vi "Main FPGA 8-axis for WPC.vi"() -> ()   [LabVIEW 2015]
uses:
  <vilib>/Motion/MotorControl/_s/nism.interpretControlRegister.stateTransition.ctl
  <vilib>/Platform/TimedLoop/XDataNode/timing_clust.ctl
  <vilib>/Platform/TimedLoop/XDataNode/nitl_modes.ctl
  <vilib>/Platform/TimedLoop/XDataNode/wakeup.ctl
  <vilib>/rvi/Emulation/niFpgaGetClockAttributes.vi
  <vilib>/rvi/Emulation/niFpgaSctlEmulationGetInTimedLoop.vi
  <vilib>/rvi/Emulation/niFpgaEmulationReportErrorSimple.vi
  Global FPGA 8-axis.vi
  <vilib>/Motion/MotorControl/_s/nism.interpretControlRegister.indexed.vi
  <vilib>/rvi/Emulation/niFpgaProcessEmulError.vi
  <vilib>/Motion/MotorControl/_s/nism.mdo.read.positionLoopSyncData.vi
  <vilib>/Motion/MotorControl/_s/nism.mdo.read.splineData.vi
  <vilib>/Motion/MotorControl/_s/nism.generateStatusRegister.indexed.vi
  <vilib>/rvi/Emulation/niFpgaCriticalErrorInLSC.vi
  <vilib>/Motion/MotorControl/_s/nism.splineInterpolation.fxp.3.index.vi
  <vilib>/Motion/MotorControl/_s/nism.mdo.handler.indexed.vi
  <vilib>/rvi/eio/common/nirviEmuTemplateMethod_errors.vi
  <vilib>/Motion/SoftMotion/Synchronization/nism.rioScan.generateSyncScan.vi
  <vilib>/Platform/TimedLoop/XDataNode/XDataNode.xnode
  <vilib>/eio/EIONode/EIONode.xnode
  <vilib>/Motion/MotorControl/NI_SoftMotion_MotorControlIP.lvlib
  <vilib>/Platform/TimedLoop/XDataNode/XDNodeRunTimeDep.lvlib
  <vilib>/Motion/SoftMotion/Synchronization/NI_SoftMotion_Synchronization.lvlib
panel:
  out "State":T1=enum."Start --> Initializing" caption="state transition"
  in  "Sync Value":bool
  in  "Sync Enable override?":bool
  out "Sync is Fault":bool
  out "Sync is Locked":bool
  in  "minimum pulse":u16=40
  # "Synchronization Loop"
  # "Control Status Loop"
  # "Notes: \n1. This VI provides the communication interface between the NI SoftMotion Engine and the LabVIEW FPGA Module. You must compile this VI for a specific FPGA target before use. After compiling, run the VI before running any of the Express VI examples. For information on moving this example to another FPGA target, refer to ni.com/info and enter info code fpgaex.\n\n2. Only use the Reset Axis button if you are unable to communicate with the axis by any other means. This button resets the device state machine and other VIs to a known state. After resetting the axis, switch the NI Scan Engine from Active Mode to Configuration Mode, then back to Active Mode, before attempting to enable the axis."
  # "(These two buttons \nare for testing\npurposes.)"
  # "Step/Direction Loop"
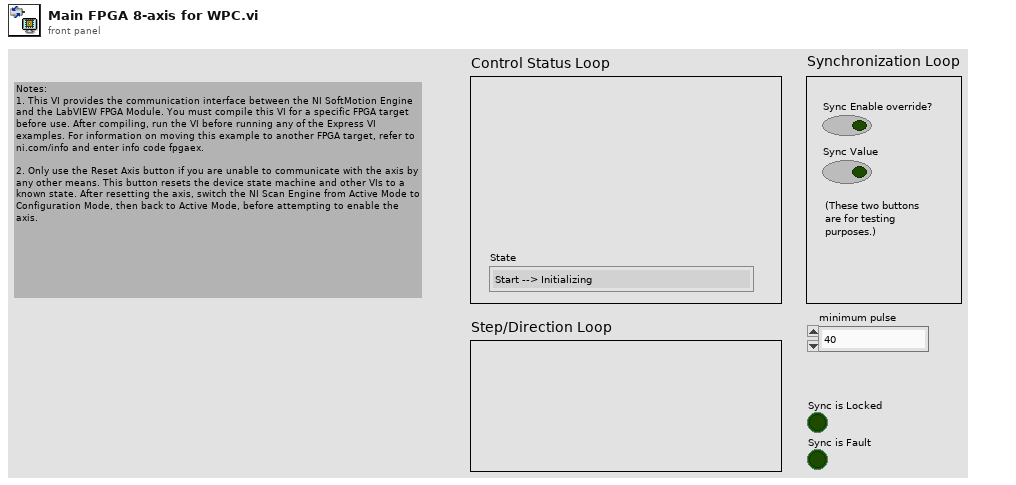
[diagram p1: front panel]
types:
  T1 = typedef "NI_SoftMotion_MotorControlIP.lvlib/nism.interpretControlRegister.stateTransition.ctl" = enum8{"Invalid", "Start --> Initializing", "Initializing --> Disabled", "Disabled --> Ready To Switch On", "Ready To Switch On --> Switched On", "Ready To Switch On --> Disable", "Switched On --> Operation Enable", "Switched On --> Ready To Switch On", "Switched On --> Disabled", "Operation Enable --> Switched On", "Operation Enable --> Ready To Switch On", "Operation Enable --> Disabled", "Fault --> Disabled", "Any --> Fault", "None"}
  T2 = typedef "NI_SoftMotion_MotorControlIP.lvlib/nism.mdo.splineData.ctl" = cluster{"spline type":T3, "traj per/spline per":u16, "spline per/traj per":fxp<+,32,0>}
  T3 = typedef "NI_SoftMotion_MotorControlIP.lvlib/nism.splineInterpolation.type.ctl" = u16
  T4 = typedef "NI_SoftMotion_Synchronization.lvlib/nism.softmotionScan.timerConfig.ctl" = cluster{"target period (clocks)":u16, "host period / target period":u16}
  T5 = typedef "NI_SoftMotion_Synchronization.lvlib/nism.softmotionScan.timerControl.ctl" = cluster{"sm scan":bool, "sm scan count":u32, "sm scan enabled":bool}
  T6 = typedef "XDNodeRunTimeDep.lvlib/timing_clust.ctl" = cluster{"Expected End [f-1]":u64, "Actual End [f-1]":u64, "Finished Late? [f-1]":bool, "Expected End [i-1]":u64, "Actual End [i-1]":u64, "Finished Late? [i-1]":bool, "Expected Start [i]":u64, "Actual Start [i]":u64, "Expected Start [f]":u64, "Actual Start [f]":u64, "Source Name":string, "Structure Name":string, "Period":i64, "Deadline":i64, "Offset":i64, "Start":i64, "Priority":i32, "Timeout":i32, "Mode":T7, "Wakeup Reason":T8, "Error":errorcluster, "Source Type":string, "Secondary Source Type":string, "Global End Time":u64, "Global Start Time":u64, "Frame Duration":u64, "Iteration Duration":u64, "Assigned CPU":i32, "I/O Scan Engine Mode":u32}
  T7 = typedef "XDNodeRunTimeDep.lvlib/nitl_modes.ctl" = enum32{"No Change", "Process missed periods, maintain original phase", "Discard missed periods, maintain original phase", "Process missed periods, ignore original phase", "Discard missed periods, ignore original phase"}
  T8 = typedef "XDNodeRunTimeDep.lvlib/wakeup.ctl" = enum32{"Normal", "Aborted", "Asynchronous wakeup", "Timing source error", "Timed loop error", "Timeout"}
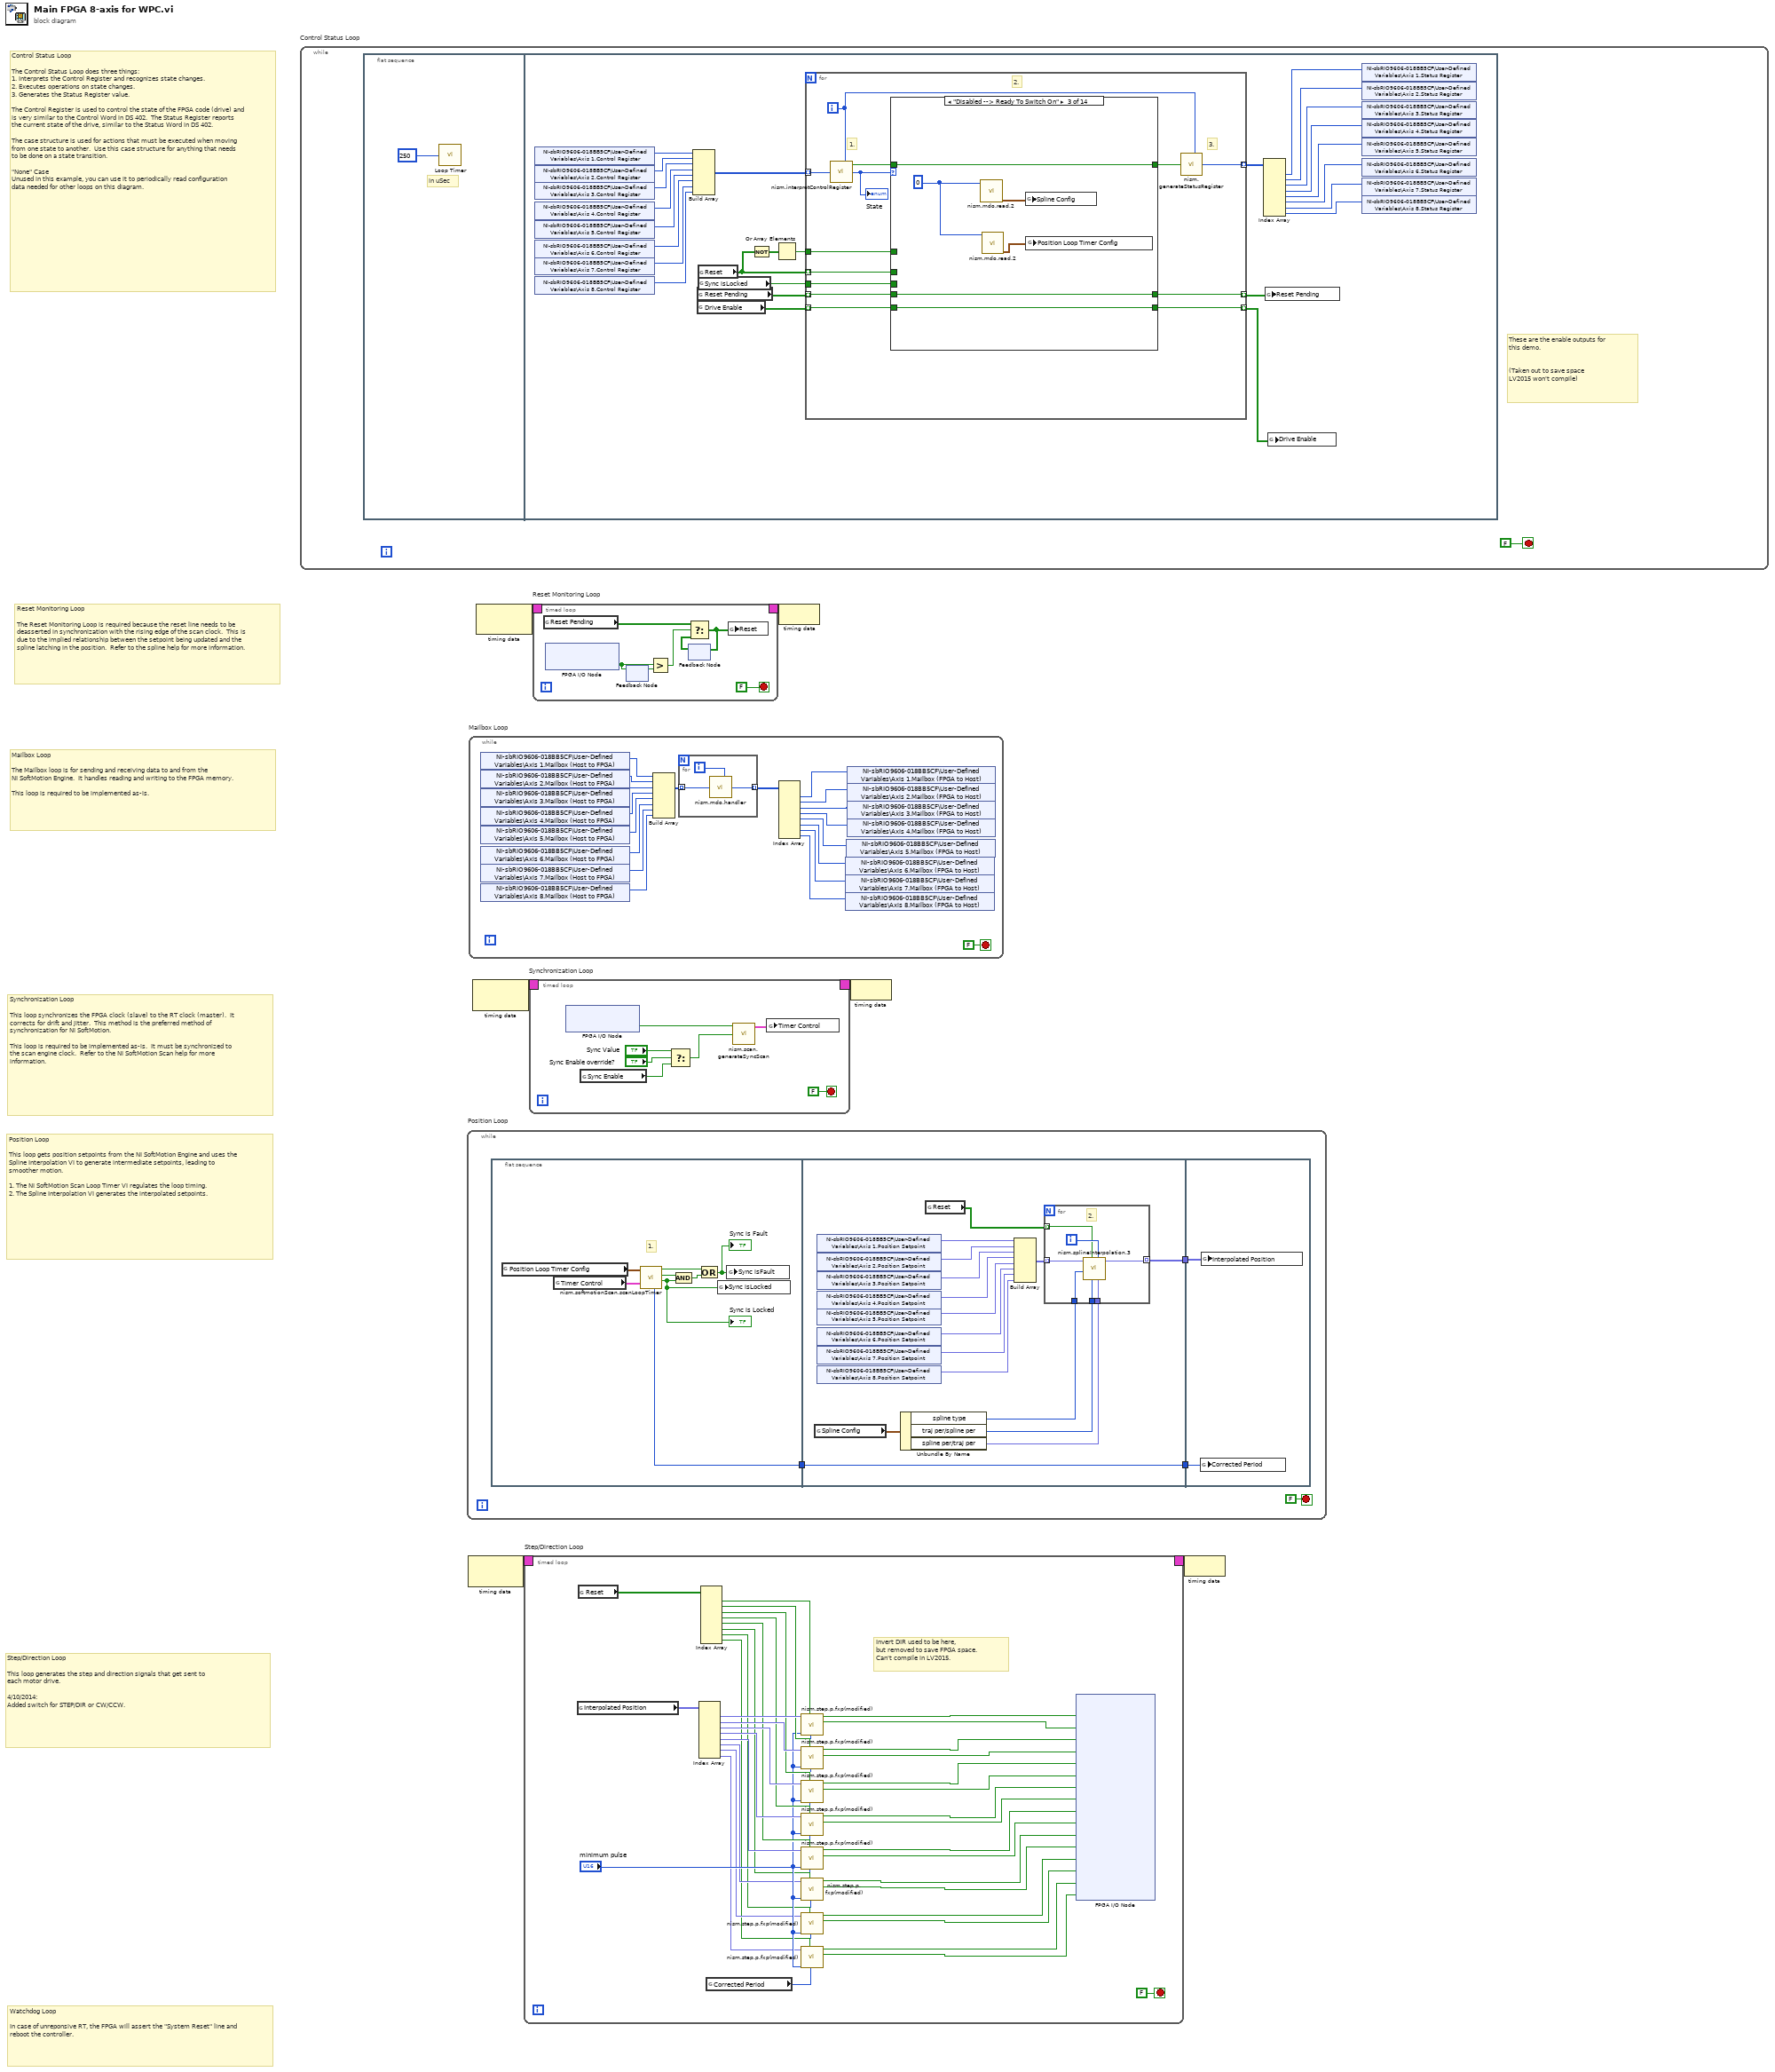
[diagram p0: block diagram]
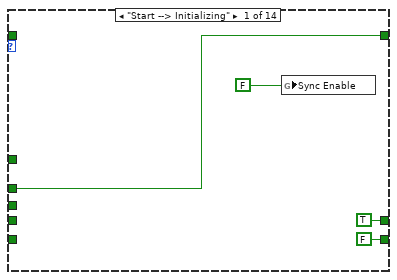
[diagram p2: hidden frame]
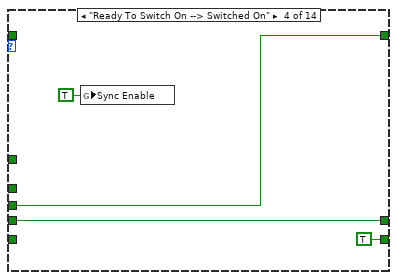
[diagram p4: hidden frame]
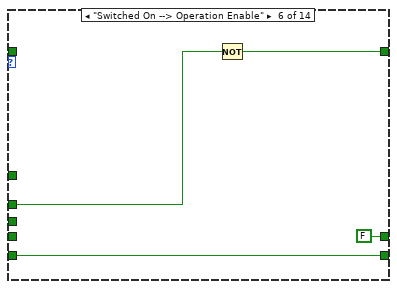
[diagram p6: hidden frame]
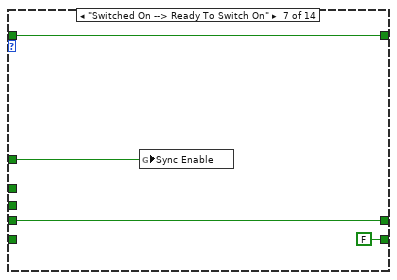
[diagram p7: hidden frame]
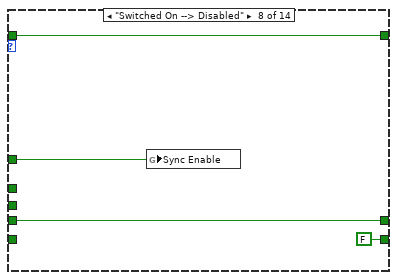
[diagram p8: hidden frame]
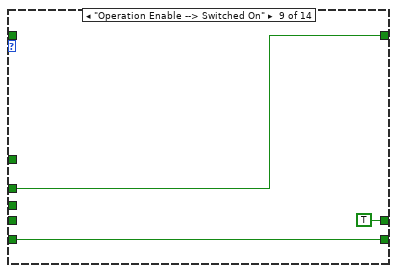
[diagram p9: hidden frame]
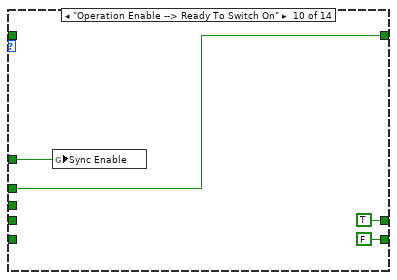
[diagram p10: hidden frame]
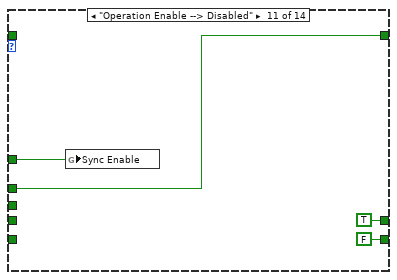
[diagram p11: hidden frame]
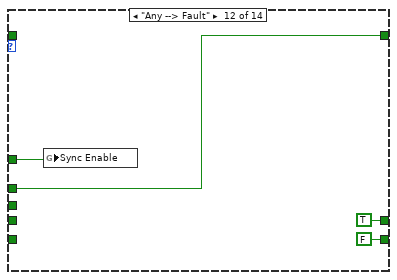
[diagram p12: hidden frame]
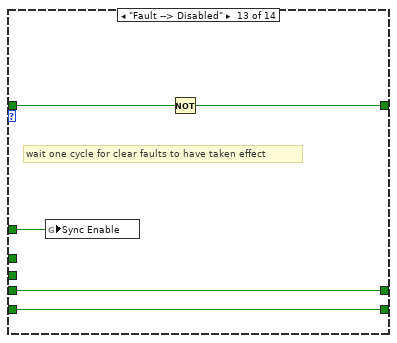
[diagram p13: hidden frame]
diagram:
  # "Watchdog Loop\n\nIn case of unreponsive RT, the FPGA will assert the \"System Reset\" line and reboot the controller."
  # "Step/Direction Loop\n\nThis loop generates the step and direction signals that get sent to \neach motor drive.\n\n4/10/2014:\nAdded switch for STEP/DIR or CW/CCW."
  # "Position Loop\n\nThis loop gets position setpoints from the NI SoftMotion Engine and uses the Spline Interpolation VI to generate intermediate setpoints, leading to smoother motion.\n\n1. The NI SoftMotion Scan Loop Timer VI regulates the loop timing. \n2. The Spline Interpolation VI generates the interpolated setpoints."
  # "Synchronization Loop\n\nThis loop synchronizes the FPGA clock (slave) to the RT clock (master).  It corrects for drift and jitter.  This method is the preferred method of synchronization for NI SoftMotion.\n\nThis loop is required to be implemented as-is.  It must be synchronized to the scan engine clock.  Refer to the NI SoftMotion Scan help for more information."
  # "Mailbox Loop\n\nThe Mailbox loop is for sending and receiving data to and from the \nNI SoftMotion Engine.  It handles reading and writing to the FPGA memory.\n\nThis loop is required to be implemented as-is."
  # "Reset Monitoring Loop\n\nThe Reset Monitoring Loop is required because the reset line needs to be deasserted in synchronization with the rising edge of the scan clock.  This is due to the implied relationship between the setpoint being updated and the spline latching in the position.  Refer to the spline help for more information."
  # "Control Status Loop\n\nThe Control Status Loop does three things:\n1. Interprets the Control Register and recognizes state changes.\n2. Executes operations on state changes.\n3. Generates the Status Register value.\n\nThe Control Register is used to control the state of the FPGA code (drive) and is very similar to the Control Word in DS 402.  The Status Register reports the current state of the drive, similar to the Status Word in DS 402.\n\nThe case structure is used for actions that must be executed when moving from one state to another.  Use this case structure for anything that needs to be done on a state transition.\n\n\"None\" Case\nUnused in this example, you can use it to periodically read configuration data needed for other loops on this diagram."
  n1 = while "Control Status Loop" {
    stop <- FALSE stop-if-true
    # "These are the enable outputs for\nthis demo.\n\n\n(Taken out to save space\nLV2015 won't compile)"
    n2 = flat-sequence {
      frame #0 {
        # "in uSec"
        n3 = call "Loop Timer"("Count(uSec)"=u8 250) -> ()  [unwired: 1 out]
      }
      frame #1 {
        n4 = shared-variable "NI-sbRIO9606-018BB5CF\\User-Defined Variables\\Axis 1.Control Register"() -> (w25:u32)  [unwired: 1 in, 1 out]
        n5 = shared-variable "NI-sbRIO9606-018BB5CF\\User-Defined Variables\\Axis 2.Control Register"() -> (w24:u32)  [unwired: 1 in, 1 out]
        n6 = shared-variable "NI-sbRIO9606-018BB5CF\\User-Defined Variables\\Axis 3.Control Register"() -> (w23:u32)  [unwired: 1 in, 1 out]
        n7 = shared-variable "NI-sbRIO9606-018BB5CF\\User-Defined Variables\\Axis 4.Control Register"() -> (w22:u32)  [unwired: 1 in, 1 out]
        n8 = shared-variable "NI-sbRIO9606-018BB5CF\\User-Defined Variables\\Axis 5.Control Register"() -> (w21:u32)  [unwired: 1 in, 1 out]
        n9 = shared-variable "NI-sbRIO9606-018BB5CF\\User-Defined Variables\\Axis 6.Control Register"() -> (w15:u32)  [unwired: 1 in, 1 out]
        n10 = shared-variable "NI-sbRIO9606-018BB5CF\\User-Defined Variables\\Axis 7.Control Register"() -> (w14:u32)  [unwired: 1 in, 1 out]
        n11 = shared-variable "NI-sbRIO9606-018BB5CF\\User-Defined Variables\\Axis 8.Control Register"() -> (w13:u32)  [unwired: 1 in, 1 out]
        n12 = Build Array(w25, w24, w23, w22, w21, w15, w14, w13) -> (w33:u32[])
        n13 = global read "Global FPGA 8-axis.vi" "Reset Pending"() -> (w28:bool[])
        n14 = global read "Global FPGA 8-axis.vi" "Drive Enable"() -> (w27:bool[])
        n15 = global read "Global FPGA 8-axis.vi" "Reset"() -> (w29:bool[])
        n16 = global read "Global FPGA 8-axis.vi" "Sync isLocked"() -> (w34:bool)
        n17 = Not(x=w29) -> (.not. x?=w31:bool[])
        n18 = Or Array Elements(Boolean array=w31) -> (logical OR=w30:bool)
        n19 = for {
          tunnel: w29 -> [w42] mode=indexing
          tunnel: w34 -> [w41]
          tunnel: w33 -> [w43] mode=indexing
          tunnel: [w40] -> w26 mode=indexing
          tunnel: [w39] -> w32 mode=indexing
          tunnel: [w38] -> w9 mode=indexing
          tunnel: w30 -> [w37]
          tunnel: w28 -> [w36] mode=indexing
          tunnel: w27 -> [w35] mode=indexing
          i -> [w44]
          # "3."
          # "2."
          # "1."
          n20 = call-poly <vilib>:"nism.interpretControlRegister.vi"("control register"=w43, "axis index"=w44) -> ("transition occurred"=w45:bool, "state transition"=w46:T1)  [unwired: 6 in]
          "State" <- w46
          n21 = case shown="\"Disabled --> Ready To Switch On\"" w46 {
            tunnel: w45 -> [_ w54 w60 _ w67 _ w75 w79 _ _ _ _ w99 _]
            tunnel: [w51 w54 w60 w62 w67 w71 w75 w79 w81 w84 w88 w92 w98 _] -> w47
            tunnel: w42 -> [w51 _ _ _ _ w70 _ _ w81 w84 w88 w92 _ _]
            tunnel: w41 -> [_ _ _ w62 _ _ _ _ _ _ _ _ _ _]
            tunnel: [TRUE ("Write.Reset Pending") w53 w56 w61 w66 FALSE ("Write.Reset Pending") w72 w76 TRUE ("Write.Reset Pending") TRUE ("Write.Reset Pending") TRUE ("Write.Reset Pending") TRUE ("Write.Reset Pending") w96 w101] -> w39
            tunnel: [FALSE ("Write.Drive Enable") w52 w55 TRUE ("Write.Drive Enable") w65 w68 FALSE ("Write.Drive Enable") FALSE ("Write.Drive Enable") w80 FALSE ("Write.Drive Enable") FALSE ("Write.Drive Enable") FALSE ("Write.Drive Enable") w95 w100] -> w38
            tunnel: w37 -> [_ _ _ _ _ _ w73 w77 _ w83 w87 w91 w97 _]
            tunnel: w36 -> [_ w53 w56 w61 w66 _ w72 w76 _ _ _ _ w96 w101]
            tunnel: w35 -> [_ w52 w55 _ w65 w68 _ _ w80 _ _ _ w95 w100]
            frame "Start --> Initializing" {
              n22 = global write "Global FPGA 8-axis.vi" "Sync Enable"(FALSE ("Sync Enable")) -> ()
            }
            frame "Initializing --> Disabled" {
            }
            frame "Disabled --> Ready To Switch On" {
              w58 = 0 ("axis index")
              n23 = call-poly <vilib>:"nism.mdo.read.2.vi"("axis index"=w58) -> ("spline"=w59:T2)  [unwired: 10 in]
              n24 = call-poly <vilib>:"nism.mdo.read.2.vi"("axis index"=w58) -> ("position loop sync"=w57:T4)  [unwired: 10 in]
              n25 = global write "Global FPGA 8-axis.vi" "Spline Config"(w59) -> ()
              n26 = global write "Global FPGA 8-axis.vi" "Position Loop Timer Config"(w57) -> ()
            }
            frame "Ready To Switch On --> Switched On" {
              n27 = global write "Global FPGA 8-axis.vi" "Sync Enable"(TRUE ("Sync Enable")) -> ()
            }
            frame "Ready To Switch On --> Disable" {
            }
            frame "Switched On --> Operation Enable" {
              n28 = Not(x=w70) -> (.not. x?=w71:bool)
            }
            frame "Switched On --> Ready To Switch On" {
              n29 = global write "Global FPGA 8-axis.vi" "Sync Enable"(w73) -> ()
            }
            frame "Switched On --> Disabled" {
              n30 = global write "Global FPGA 8-axis.vi" "Sync Enable"(w77) -> ()
            }
            frame "Operation Enable --> Switched On" {
            }
            frame "Operation Enable --> Ready To Switch On" {
              n31 = global write "Global FPGA 8-axis.vi" "Sync Enable"(w83) -> ()
            }
            frame "Operation Enable --> Disabled" {
              n32 = global write "Global FPGA 8-axis.vi" "Sync Enable"(w87) -> ()
            }
            frame "Any --> Fault" {
              n33 = global write "Global FPGA 8-axis.vi" "Sync Enable"(w91) -> ()
            }
            frame "Fault --> Disabled" {
              # "wait one cycle for clear faults to have taken effect"
              n34 = global write "Global FPGA 8-axis.vi" "Sync Enable"(w97) -> ()
              n35 = Not(x=w99) -> (.not. x?=w98:bool)
            }
            frame "None", Default {
            }
          }
          n36 = call-poly <vilib>:"nism.generateStatusRegister.vi"("transition success"=w47, "axis index"=w44) -> ("status register"=w40:u32)  [unwired: 7 in]
        }
        n37 = Index Array(array=w26) -> (element #1=w20:u32, element #2=w19:u32, element #3=w18:u32, element #4=w17:u32, element #5=w16:u32, element #6=w12:u32, element #7=w11:u32, element #8=w10:u32)  [unwired: 8 in]
        n38 = global write "Global FPGA 8-axis.vi" "Reset Pending"(w32) -> ()
        n39 = global write "Global FPGA 8-axis.vi" "Drive Enable"(w9) -> ()
        n40 = shared-variable "NI-sbRIO9606-018BB5CF\\User-Defined Variables\\Axis 1.Status Register"(w20) -> ()  [unwired: 1 in, 1 out]
        n41 = shared-variable "NI-sbRIO9606-018BB5CF\\User-Defined Variables\\Axis 2.Status Register"(w19) -> ()  [unwired: 1 in, 1 out]
        n42 = shared-variable "NI-sbRIO9606-018BB5CF\\User-Defined Variables\\Axis 3.Status Register"(w18) -> ()  [unwired: 1 in, 1 out]
        n43 = shared-variable "NI-sbRIO9606-018BB5CF\\User-Defined Variables\\Axis 4.Status Register"(w17) -> ()  [unwired: 1 in, 1 out]
        n44 = shared-variable "NI-sbRIO9606-018BB5CF\\User-Defined Variables\\Axis 5.Status Register"(w16) -> ()  [unwired: 1 in, 1 out]
        n45 = shared-variable "NI-sbRIO9606-018BB5CF\\User-Defined Variables\\Axis 6.Status Register"(w12) -> ()  [unwired: 1 in, 1 out]
        n46 = shared-variable "NI-sbRIO9606-018BB5CF\\User-Defined Variables\\Axis 7.Status Register"(w11) -> ()  [unwired: 1 in, 1 out]
        n47 = shared-variable "NI-sbRIO9606-018BB5CF\\User-Defined Variables\\Axis 8.Status Register"(w10) -> ()  [unwired: 1 in, 1 out]
      }
    }
  }
  n48 = while "Position Loop" {
    stop <- FALSE stop-if-true
    n49 = flat-sequence {
      tunnel: [w106] -> w102
      tunnel: [w123] -> w104
      tunnel: [w122] -> w103
      tunnel: w102 -> [w122]
      tunnel: w104 -> [w137]
      tunnel: w103 -> [w138]
      frame #0 {
        # "1."
        n50 = global read "Global FPGA 8-axis.vi" "Position Loop Timer Config"() -> (w108:T4)
        n51 = global read "Global FPGA 8-axis.vi" "Timer Control"() -> (w107:T5)
        n52 = call <vilib>:"nism.softmotionScan.scanLoopTimer.vi"("timer control"=w107, "timer config"=w108) -> ("scan running?"=w110:bool, "finished late?"=w112:bool, "fault occurred?"=w113:bool, "corrected period"=w106:u16)  [unwired: 5 in, 1 out]
        "Sync is Locked" <- w110
        n53 = Compound Arithmetic op=AND(w112, w110) -> (w111:bool)
        n54 = Compound Arithmetic op=OR(w113, w111) -> (w109:bool)
        "Sync is Fault" <- w109
        n55 = global write "Global FPGA 8-axis.vi" "Sync isLocked"(w110) -> ()
        n56 = global write "Global FPGA 8-axis.vi" "Sync isFault"(w109) -> ()
      }
      frame #1 {
        n57 = global read "Global FPGA 8-axis.vi" "Spline Config"() -> (w125:T2)
        n58 = shared-variable "NI-sbRIO9606-018BB5CF\\User-Defined Variables\\Axis 1.Position Setpoint"() -> (w121:fxp<+/-,64,32>)  [unwired: 1 in, 1 out]
        n59 = shared-variable "NI-sbRIO9606-018BB5CF\\User-Defined Variables\\Axis 2.Position Setpoint"() -> (w120:fxp<+/-,64,32>)  [unwired: 1 in, 1 out]
        n60 = shared-variable "NI-sbRIO9606-018BB5CF\\User-Defined Variables\\Axis 3.Position Setpoint"() -> (w119:fxp<+/-,64,32>)  [unwired: 1 in, 1 out]
        n61 = shared-variable "NI-sbRIO9606-018BB5CF\\User-Defined Variables\\Axis 4.Position Setpoint"() -> (w118:fxp<+/-,64,32>)  [unwired: 1 in, 1 out]
        n62 = shared-variable "NI-sbRIO9606-018BB5CF\\User-Defined Variables\\Axis 5.Position Setpoint"() -> (w117:fxp<+/-,64,32>)  [unwired: 1 in, 1 out]
        n63 = shared-variable "NI-sbRIO9606-018BB5CF\\User-Defined Variables\\Axis 6.Position Setpoint"() -> (w116:fxp<+/-,64,32>)  [unwired: 1 in, 1 out]
        n64 = shared-variable "NI-sbRIO9606-018BB5CF\\User-Defined Variables\\Axis 7.Position Setpoint"() -> (w115:fxp<+/-,64,32>)  [unwired: 1 in, 1 out]
        n65 = shared-variable "NI-sbRIO9606-018BB5CF\\User-Defined Variables\\Axis 8.Position Setpoint"() -> (w114:fxp<+/-,64,32>)  [unwired: 1 in, 1 out]
        n66 = Unbundle By Name(w125) -> ("spline type"=w129:T3, "traj per/spline per"=w128:u16, "spline per/traj per"=w127:fxp<+,32,0>)
        n67 = global read "Global FPGA 8-axis.vi" "Reset"() -> (w124:bool[])
        n68 = Build Array(w121, w120, w119, w118, w117, w116, w115, w114) -> (w126:fxp<+/-,64,32>[])
        n69 = for {
          tunnel: w129 -> [w136]
          tunnel: w128 -> [w135]
          tunnel: w127 -> [w134]
          tunnel: w124 -> [w131] mode=indexing
          tunnel: w126 -> [w133] mode=indexing
          tunnel: [w130] -> w123 mode=indexing
          i -> [w132]
          # "2."
          n70 = call-poly <vilib>:"nism.splineInterpolation.3.vi"("1 / calls per sample"=w134, "index"=w132, "calls per sample"=w135, "reset"=w131, "spline type"=w136, "x"=w133) -> ("xi"=w130:fxp<+/-,64,32>)  [unwired: 4 in, 1 out]
        }
      }
      frame #2 {
        n71 = global write "Global FPGA 8-axis.vi" "Corrected Period"(w138) -> ()
        n72 = global write "Global FPGA 8-axis.vi" "Interpolated Position"(w137) -> ()
      }
    }
  }
  n73 = node-c288() -> (w6:T6)  [unwired: 1 in]
  n74 = while "Mailbox Loop" {
    stop <- FALSE stop-if-true
    n75 = shared-variable "NI-sbRIO9606-018BB5CF\\User-Defined Variables\\Axis 1.Mailbox (Host to FPGA)"() -> (w154:u64)  [unwired: 1 in, 1 out]
    n76 = shared-variable "NI-sbRIO9606-018BB5CF\\User-Defined Variables\\Axis 2.Mailbox (Host to FPGA)"() -> (w153:u64)  [unwired: 1 in, 1 out]
    n77 = shared-variable "NI-sbRIO9606-018BB5CF\\User-Defined Variables\\Axis 3.Mailbox (Host to FPGA)"() -> (w152:u64)  [unwired: 1 in, 1 out]
    n78 = shared-variable "NI-sbRIO9606-018BB5CF\\User-Defined Variables\\Axis 4.Mailbox (Host to FPGA)"() -> (w151:u64)  [unwired: 1 in, 1 out]
    n79 = shared-variable "NI-sbRIO9606-018BB5CF\\User-Defined Variables\\Axis 5.Mailbox (Host to FPGA)"() -> (w150:u64)  [unwired: 1 in, 1 out]
    n80 = shared-variable "NI-sbRIO9606-018BB5CF\\User-Defined Variables\\Axis 6.Mailbox (Host to FPGA)"() -> (w144:u64)  [unwired: 1 in, 1 out]
    n81 = shared-variable "NI-sbRIO9606-018BB5CF\\User-Defined Variables\\Axis 7.Mailbox (Host to FPGA)"() -> (w143:u64)  [unwired: 1 in, 1 out]
    n82 = shared-variable "NI-sbRIO9606-018BB5CF\\User-Defined Variables\\Axis 8.Mailbox (Host to FPGA)"() -> (w142:u64)  [unwired: 1 in, 1 out]
    n83 = Build Array(w154, w153, w152, w151, w150, w144, w143, w142) -> (w156:u64[])
    n84 = for {
      tunnel: w156 -> [w160] mode=indexing
      tunnel: [w159] -> w155 mode=indexing
      i -> [w158]
      n85 = call-poly <vilib>:"nism.mdo.handler.vi"("mbox (host to fpga)"=w160, "axis index"=w158) -> ("mbox (fpga to host)"=w159:u64)  [unwired: 7 in]
    }
    n86 = Index Array(array=w155) -> (element #1=w149:u64, element #2=w148:u64, element #3=w147:u64, element #4=w146:u64, element #5=w145:u64, element #6=w141:u64, element #7=w140:u64, element #8=w139:u64)  [unwired: 8 in]
    n87 = shared-variable "NI-sbRIO9606-018BB5CF\\User-Defined Variables\\Axis 6.Mailbox (FPGA to Host)"(w141) -> ()  [unwired: 1 in, 1 out]
    n88 = shared-variable "NI-sbRIO9606-018BB5CF\\User-Defined Variables\\Axis 7.Mailbox (FPGA to Host)"(w140) -> ()  [unwired: 1 in, 1 out]
    n89 = shared-variable "NI-sbRIO9606-018BB5CF\\User-Defined Variables\\Axis 8.Mailbox (FPGA to Host)"(w139) -> ()  [unwired: 1 in, 1 out]
    n90 = shared-variable "NI-sbRIO9606-018BB5CF\\User-Defined Variables\\Axis 5.Mailbox (FPGA to Host)"(w145) -> ()  [unwired: 1 in, 1 out]
    n91 = shared-variable "NI-sbRIO9606-018BB5CF\\User-Defined Variables\\Axis 1.Mailbox (FPGA to Host)"(w149) -> ()  [unwired: 1 in, 1 out]
    n92 = shared-variable "NI-sbRIO9606-018BB5CF\\User-Defined Variables\\Axis 2.Mailbox (FPGA to Host)"(w148) -> ()  [unwired: 1 in, 1 out]
    n93 = shared-variable "NI-sbRIO9606-018BB5CF\\User-Defined Variables\\Axis 3.Mailbox (FPGA to Host)"(w147) -> ()  [unwired: 1 in, 1 out]
    n94 = shared-variable "NI-sbRIO9606-018BB5CF\\User-Defined Variables\\Axis 4.Mailbox (FPGA to Host)"(w146) -> ()  [unwired: 1 in, 1 out]
  }
  n95 = node-c288() -> (w4:T6)  [unwired: 1 in]
  n96 = node-c288() -> (w2:T6)  [unwired: 1 in]
  n97 = timed-loop "Step/Direction Loop" {
    timing: w6 -> [_]
    timing-out: [_] -> w5
    stop <- FALSE stop-if-true
    # "Invert DIR used to be here,\nbut removed to save FPGA space.\nCan't compile in LV2015."
    n98 = global read "Global FPGA 8-axis.vi" "Interpolated Position"() -> (w196:fxp<+/-,64,32>[])
    n99 = global read "Global FPGA 8-axis.vi" "Reset"() -> (w190:bool[])
    n100 = Index Array(array=w196) -> (element #1=w195:fxp<+/-,64,32>, element #2=w194:fxp<+/-,64,32>, element #3=w193:fxp<+/-,64,32>, element #4=w192:fxp<+/-,64,32>, element #5=w191:fxp<+/-,64,32>, element #6=w183:fxp<+/-,64,32>, element #7=w182:fxp<+/-,64,32>, element #8=w181:fxp<+/-,64,32>)  [unwired: 8 in]
    n101 = Index Array(array=w190) -> (element #1=w189:bool, element #2=w188:bool, element #3=w187:bool, element #4=w186:bool, element #5=w185:bool, element #6=w180:bool, element #7=w179:bool, element #8=w178:bool)  [unwired: 8 in]
    n102 = global read "Global FPGA 8-axis.vi" "Corrected Period"() -> (w177:u16)
    n103 = call "nism.step.p.fxp(modified).vi"("calls per sample"=w177, "reset"=w189, "minimum pulse"="minimum pulse", "position setpoint"=w195) -> ("step"=w175:bool, "direction"=w176:bool)  [unwired: 4 in, 2 out]
    n104 = call "nism.step.p.fxp(modified).vi"("calls per sample"=w177, "reset"=w188, "minimum pulse"="minimum pulse", "position setpoint"=w194) -> ("step"=w173:bool, "direction"=w174:bool)  [unwired: 4 in, 2 out]
    n105 = call "nism.step.p.fxp(modified).vi"("calls per sample"=w177, "reset"=w187, "minimum pulse"="minimum pulse", "position setpoint"=w193) -> ("step"=w171:bool, "direction"=w172:bool)  [unwired: 4 in, 2 out]
    n106 = call "nism.step.p.fxp(modified).vi"("calls per sample"=w177, "reset"=w186, "minimum pulse"="minimum pulse", "position setpoint"=w192) -> ("step"=w169:bool, "direction"=w170:bool)  [unwired: 4 in, 2 out]
    n107 = call "nism.step.p.fxp(modified).vi"("calls per sample"=w177, "reset"=w185, "minimum pulse"="minimum pulse", "position setpoint"=w191) -> ("step"=w167:bool, "direction"=w168:bool)  [unwired: 4 in, 2 out]
    n108 = call "nism.step.p.fxp(modified).vi"("calls per sample"=w177, "reset"=w180, "minimum pulse"="minimum pulse", "position setpoint"=w183) -> ("step"=w165:bool, "direction"=w166:bool)  [unwired: 4 in, 2 out]
    n109 = call "nism.step.p.fxp(modified).vi"("calls per sample"=w177, "reset"=w179, "minimum pulse"="minimum pulse", "position setpoint"=w182) -> ("step"=w163:bool, "direction"=w164:bool)  [unwired: 4 in, 2 out]
    n110 = call "nism.step.p.fxp(modified).vi"("calls per sample"=w177, "reset"=w178, "minimum pulse"="minimum pulse", "position setpoint"=w181) -> ("step"=w161:bool, "direction"=w162:bool)  [unwired: 4 in, 2 out]
    n111 = xnode "FPGA I/O Node"("RMC/DIO46"=w176, "RMC/DIO47"=w175, "RMC/DIO14"=w174, "RMC/DIO63"=w173, "RMC/DIO95"=w172, "RMC/DIO31"=w171, "RMC/DIO30"=w170, "RMC/DIO45"=w169, "RMC/DIO77"=w168, "RMC/DIO44"=w167, "RMC/DIO12"=w166, "RMC/DIO94"=w165, "RMC/DIO93"=w164, "RMC/DIO29"=w163, "RMC/DIO28"=w162, "RMC/DIO43"=w161) -> ()  [unwired: 16 in, 16 out]
  }
  n112 = timed-loop "Synchronization Loop" {
    timing: w4 -> [_]
    timing-out: [_] -> w3
    stop <- FALSE stop-if-true
    n113 = xnode "FPGA I/O Node"() -> ("Scan Clock"=w204:bool)  [unwired: 1 in, 1 out]
    n114 = global read "Global FPGA 8-axis.vi" "Sync Enable"() -> (w203:bool)
    n115 = Select(t="Sync Value", s="Sync Enable override?", f=w203) -> (s? t:f=w200:bool)
    n116 = call-poly <vilib>:"nism.scan.generateSyncScan.vi"("scan enable?"=w200, "scan clock"=w204) -> ("timer control"=w205:T5)  [unwired: 3 in]
    n117 = global write "Global FPGA 8-axis.vi" "Timer Control"(w205) -> ()
  }
  n118 = timed-loop "Reset Monitoring Loop" {
    timing: w2 -> [_]
    timing-out: [_] -> w1
    stop <- FALSE stop-if-true
    n119 = global read "Global FPGA 8-axis.vi" "Reset Pending"() -> (w211:bool[])
    n120 = xnode "FPGA I/O Node"() -> ("Scan Clock"=w210:bool)  [unwired: 1 in, 1 out]
    n121 = feedback-in #1(w210) -> ()
    n122 = feedback #1() -> (w209:bool)  [unwired: 1 in]
    n123 = Greater?(x=w210, y=w209) -> (0:w215:bool)
    n124 = feedback #2() -> (w214:bool[])  [unwired: 1 in]
    n125 = Select(t=w211, s=w215, f=w214) -> (s? t:f=w212:bool[])
    n126 = feedback-in #2(w212) -> ()
    n127 = global write "Global FPGA 8-axis.vi" "Reset"(w212) -> ()
  }
  n128 = node-c288(w1) -> ()
  n129 = node-c288(w3) -> ()
  n130 = node-c288(w5) -> ()
